vi "ReadTubeCorrnFile.vi"(11 "PathToFile":path) -> (2 "F-CompArray":dbl[][](array[numeric]))   [LabVIEW 2011]
panel:
  out "FileContents":string
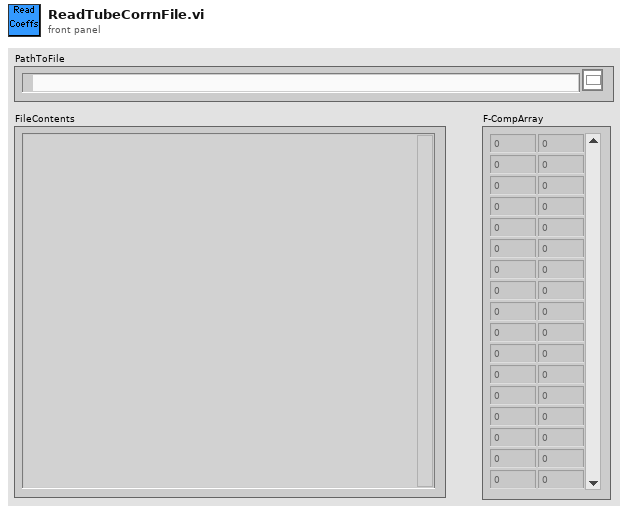
[diagram p1: front panel]
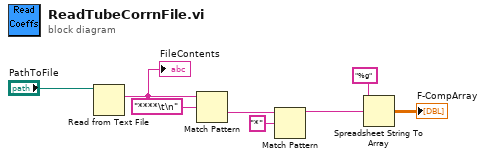
[diagram p0: block diagram]
diagram:
  n1 = Read from Text File(file (use dialog)="PathToFile") -> (text=w8:string)  [unwired: 3 in, 3 out]
  "FileContents" <- w8
  n2 = Match Pattern(string=w8, regular expression="****\t\n") -> (after substring=w3:string)  [unwired: 1 in, 3 out]
  n3 = Match Pattern(string=w3, regular expression="*") -> (before substring=w1:string)  [unwired: 1 in, 3 out]
  n4 = Spreadsheet String To Array(format string="%g", spreadsheet string=w1) -> (array=→"F-CompArray":dbl[][])  [unwired: 2 in]
